vi "Double_Integrador_BIG (SubVI).vi"(6 "Mode":bool, 7 "Iteration":i32, 8 "Int_2_k_1":dbl, 9 "Int_1_k_1":dbl, 10 "Value":i32, 11 "Speed":dbl) -> (0 "Integral 2":dbl, 1 "Integral 1":dbl)   [LabVIEW 2017]
panel:
  # "VI que calcula el doble integrador de una constante. \nUsado en el calculo de la señal de referencia para el control de los motores.\nWRO2018 @ Steve Mena Navarro."
  # "Entradas: \nInt_1k_1: Valor del primer integrador en la iteración anterior.\nSpeed: Señal a integrar\nValue: Valor final del integrador.\nInt_2_k_1: Valor del segundo integrador interación anterior.\nIteration: Número de iteración.\n\nSalidas: \nIntegral 1: Valor del primer integrador en interación actual.\nIntegral2 : Valor del segundo integrador en iteración actual."
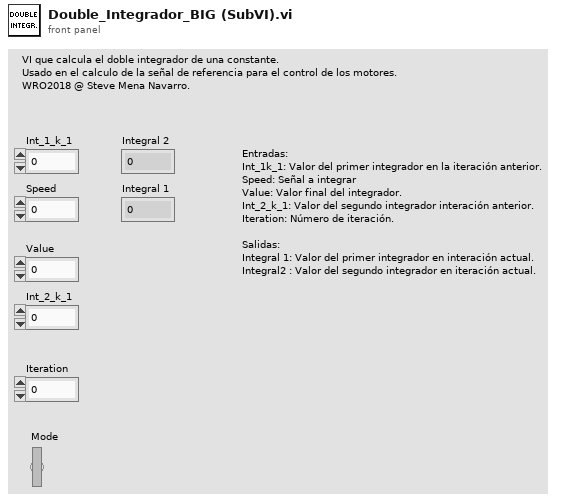
[diagram p1: front panel]
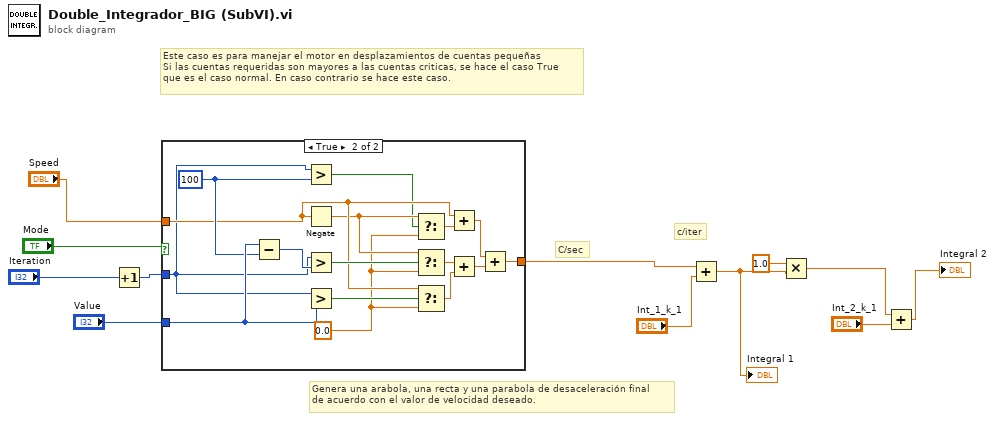
[diagram p0: block diagram]
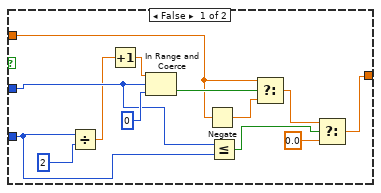
[diagram p2: hidden frame]
diagram:
  # "c/iter"
  # "C/sec"
  # "Este caso es para manejar el motor en desplazamientos de cuentas pequeñas\nSi las cuentas requeridas son mayores a las cuentas criticas, se hace el caso True\nque es el caso normal. En caso contrario se hace este caso."
  # "Genera una arabola, una recta y una parabola de desaceleración final\nde acuerdo con el valor de velocidad deseado."
  n1 = Increment(x="Iteration") -> (x+1=w1:i32)
  n2 = case shown="True" "Mode" {
    tunnel: "Value" -> [w15 w41]
    tunnel: w1 -> [w17 w26]
    tunnel: "Speed" -> [w21 w36]
    tunnel: [w19 w35] -> w5
    frame False {
      n3 = Divide(x=w15, y=2) -> (x/y=w13:dbl)
      n4 = Increment(x=w13) -> (x+1=w14:dbl)
      n5 = In Range and Coerce(upper limit=w14, x=w17, lower limit=u32 0) -> (In Range?=w23:bool)  [unwired: 1 out]
      n6 = Negate(x=w21) -> (-x=w22:dbl)
      n7 = Less Or Equal?(x=w17, y=w15) -> (x <= y?=w16:bool)
      n8 = Select(t=w21, s=w23, f=w22) -> (s? t:f=w20:dbl)
      n9 = Select(t=w20, s=w16, f=0.0) -> (s? t:f=w19:dbl)
    }
    frame True {
      w27 = 0.0
      w39 = 100 ("y")
      n10 = Subtract(x=w41, y=w39) -> (x-y=w40:i32)
      n11 = Greater?(x=w26, y=w39) -> (0:w28:bool)
      n12 = Negate(x=w36) -> (-x=w29:dbl)
      n13 = Greater?(x=w26, y=w40) -> (0:w38:bool)
      n14 = Greater?(x=w26, y=w41) -> (0:w37:bool)
      n15 = Select(t=w29, s=w28, f=w27) -> (s? t:f=w30:dbl)
      n16 = Select(t=w29, s=w38, f=w27) -> (s? t:f=w31:dbl)
      n17 = Select(t=w36, s=w37, f=w27) -> (s? t:f=w32:dbl)
      n18 = Add(x=w36, y=w30) -> (x+y=w33:dbl)
      n19 = Add(x=w31, y=w32) -> (x+y=w34:dbl)
      n20 = Add(x=w33, y=w34) -> (x+y=w35:dbl)
    }
  }
  n21 = Add(x=w5, y="Int_1_k_1") -> (x+y=w6:dbl)
  "Integral 1" <- w6
  n22 = Multiply(x=1.0, y=w6) -> (x*y=w7:dbl)
  n23 = Add(x=w7, y="Int_2_k_1") -> (x+y=→"Integral 2":dbl)
